vi "GPIB-WriteRead.vi"(2 "# bytes\nto read":i32=200, 4 "Characters to Write":string) -> (1 "Write error out":errorcluster, 3 "Characters Read":string)   [LabVIEW 2019]
panel:
  out "Read error out":errorcluster
  in  "Read":bool=TRUE
  in  "Write":bool=TRUE
  # "Select  the GPIB address of the device, choose Read or Write or both, type in the characters to be written, and run the VI. If you choose both Read and Write, the VI will write to the device first, then read from the device.  Before using this VI, you should consider initializing the bus with the \"GPIB Initialization\" function."
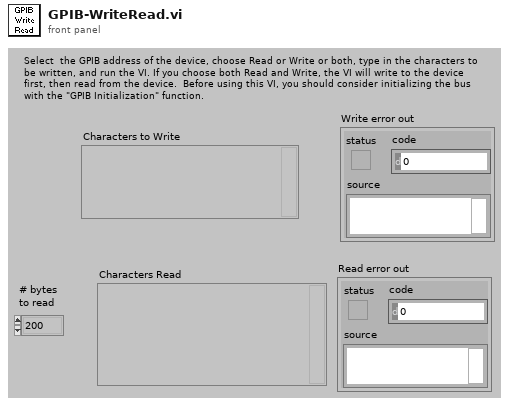
[diagram p1: front panel]
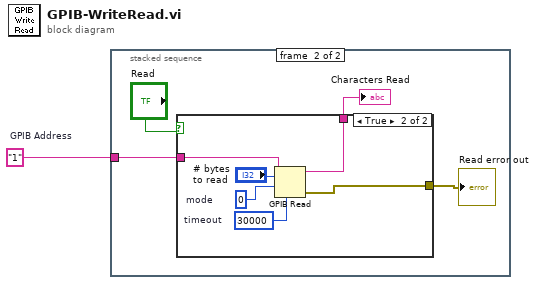
[diagram p0: block diagram]
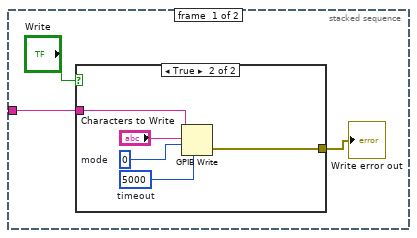
[diagram p2: hidden frame]
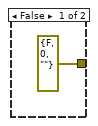
[diagram p3: hidden frame]
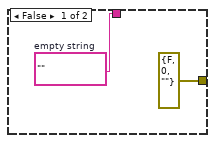
[diagram p4: hidden frame]
diagram:
  w1 = "1"  # GPIB Address
  n1 = stacked-sequence {
    tunnel: w1 -> [w4 w14]
    frame #0 {
      n2 = case shown="True" "Write" {
        tunnel: w4 -> [_ w8]
        tunnel: [errorcluster {"status"=FALSE, "code"=0, "source"=""} ("error out") w6] -> w2
        frame False {
        }
        frame True {
          w10 = 0  # mode
          w7 = u32 5000  # timeout
          n3 = GPIB Write(0:w8, 1:"Characters to Write", 2:w10, 4:w7) -> (6:w6:errorcluster)  [unwired: 1 in, 1 out]
        }
      }
      "Write error out" <- w2
    }
    frame #1 {
      n4 = case shown="True" "Read" {
        tunnel: [w16 w19] -> w12
        tunnel: [errorcluster {"status"=FALSE, "code"=0, "source"=""} ("error out") w17] -> w11
        tunnel: w14 -> [_ w21]
        frame False {
          w16 = ""  # empty string
        }
        frame True {
          w18 = u32 30000  # timeout
          w22 = 0  # mode
          n5 = GPIB Read(0:w21, 1:"# bytes\nto read", 2:w22, 4:w18) -> (5:w19:string, 7:w17:errorcluster)  [unwired: 1 in, 1 out]
        }
      }
      "Characters Read" <- w12
      "Read error out" <- w11
    }
  }
